vi "subVI_1.vi"(9 "String":string, 10 "Array":string[](array[string]), 11 "Numeric in":i32) -> (2 "Boolean":bool, 3 "Numeric out":i32)   [LabVIEW 2016]
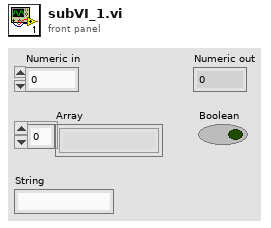
[diagram p1: front panel]
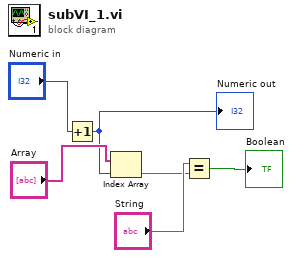
[diagram p0: block diagram]
diagram:
  n1 = Increment(x="Numeric in") -> (x+1=w5:i32)
  "Numeric out" <- w5
  n2 = Index Array(array="Array", index=w5) -> (element=w1:string)
  n3 = Equal?(x="String", y=w1) -> (x = y?=→"Boolean":bool)
